vi "NotifyOwner(SelfTermination).vi"(8 "error in (no error)":errorcluster, 11 "SMO in":refnum<class "SMO.lvclass">) -> (0 "error out":errorcluster, 3 "SMO out":refnum<class "SMO.lvclass">)   [LabVIEW 2019, in "SMO.lvclass"]
doc: "JKI State Machine Objects (SMO) 1.3.0.56\nJKI - JKI\nCopyright (c) 2017, JKI"
uses:
  SMO.lvclass
  Support/Attribute.Owner/Attribute.Owner.lvclass
  C:/Users/Patrick/Documents/GitHub/Test (LV2019)/lv-venv/lv.lib/vi.lib/JKI/JKI SMO/Support/Attribute/Attribute.lvclass
  Support/Attribute/Attribute.lvclass
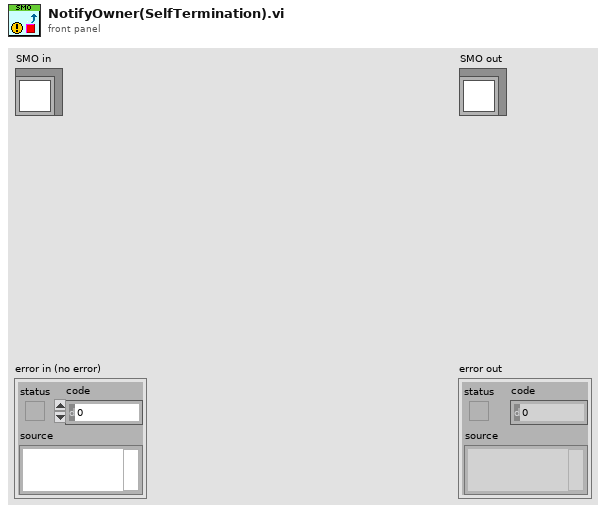
[diagram p1: front panel]
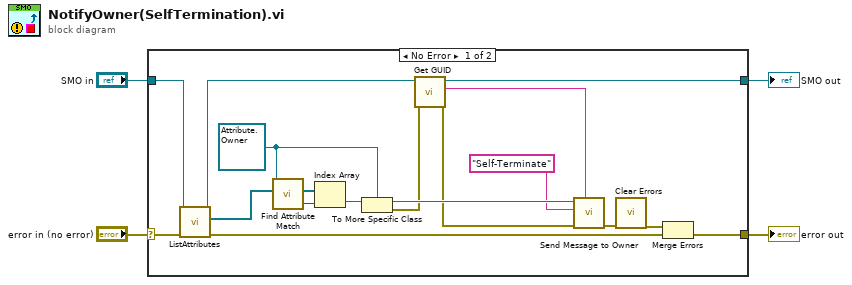
[diagram p0: block diagram]
diagram:
  n1 = case shown="No Error" "error in (no error)" {
    selector: "error in (no error)" -> [w20 w24]
    tunnel: [w12 w24] -> w3
    tunnel: [w10 w23] -> w1
    tunnel: "SMO in" -> [w21 w23]
    frame No Error {
      w11 = refnum<class "Attribute.Owner.lvclass"> refnum ("Attribute.Owner.lvclass")
      n2 = call "ListAttributes.vi"("error in (no error)"=w20, "SMO in"=w21) -> ("error out"=w13:errorcluster, "[Attributes]"=w22:refnum<class "Attribute.lvclass">[], "SMO out"=w8:refnum<class "SMO.lvclass">)  [unwired: 7 in]
      n3 = call "Find Attribute Match.vi"("Attributes"=w22, "Attribute in"=w11) -> ("Matched index"=w18:i32, "Attributes dup"=w19:refnum<class "Attribute.lvclass">[])  [unwired: 7 in, 1 out]
      n4 = Index Array(array=w19, index=w18) -> (element=w17:refnum<class "Attribute.lvclass">)
      n5 = To More Specific Class(target class=w11, reference=w17) -> (specific class reference=w16:refnum<class "Attribute.Owner.lvclass">, error out=w7:errorcluster)  [unwired: 1 in]
      n6 = call "Get GUID.vi"("error in (no error)"=w7, "SMO"=w8) -> ("error out"=w9:errorcluster, "GUID"=w6:string, "SMO out"=w10:refnum<class "SMO.lvclass">)  [unwired: 7 in]
      n7 = call "Send Message to Owner.vi"("GUID"=w6, "error in (no error)"=w9, "Message"="Self-Terminate", "Attribute.Owner in"=w16) -> ("error out"=w15:errorcluster)  [unwired: 6 in, 1 out]
      n8 = call <vilib>:"Clear Errors.vi"("error in (no error)"=w15) -> ("error out"=w14:errorcluster)  [unwired: 5 in, 1 out]
      n9 = Merge Errors(w14, w13) -> (w12:errorcluster)
    }
    frame Error {
    }
  }
  "error out" <- w3
  "SMO out" <- w1
